vi "Add Header LV2012 NIVerified.vi"() -> ()   [LabVIEW 2012]
doc: "This example describes how to add a simple header to a spreadsheet file built with the Write to Spreadsheet File VI."
uses:
  <vilib>/Utility/file.llb/Write To Spreadsheet File (string).vi
panel:
  in  "stop":bool
  in  "Path":path
  # "Overview: This example describes how to add a simple header to a spreadsheet file built with the Write to Spreadsheet File VI.\n\nRequirements: LabVIEW 2012 (or compatible).\n\nInstructions\n1. Select a file path.\n2. Run this VI."
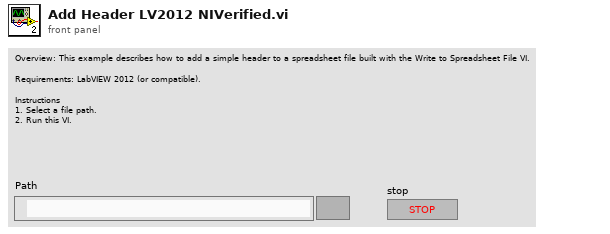
[diagram p1: front panel]
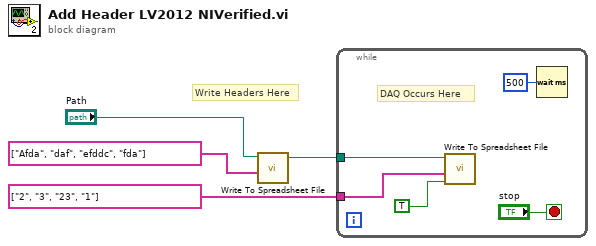
[diagram p0: block diagram]
diagram:
  # "Write Headers Here"
  n1 = call-poly <vilib>:"Write To Spreadsheet File.vi"("1D data"=string[] ["Afda", "daf", "efddc", "fda"], "file path (dialog if empty)"="Path") -> ("new file path (Not A Path if cancelled)"=w1:path)  [unwired: 4 in, 2 out]
  n2 = while {
    tunnel: string[] ["2", "3", "23", "1"] -> [w9]
    tunnel: w1 -> [w5]
    stop <- "stop" stop-if-true
    # "DAQ Occurs Here"
    n3 = call-poly <vilib>:"Write To Spreadsheet File.vi"("append to file? (new file:F)"=TRUE, "1D data"=w9, "file path (dialog if empty)"=w5) -> ()  [unwired: 3 in, 3 out]
    n4 = Wait (ms)(milliseconds to wait=u32 500) -> ()  [unwired: 1 out]
  }
